vi "Load.vi"(8 "error in (no error)":errorcluster, 9 "Automatic?":bool, 10 "configuration file path":path, 11 "SettingsFile in":refnum<class "SettingsFile.lvclass">) -> (0 "error out":errorcluster, 3 "SettingsFile out":refnum<class "SettingsFile.lvclass">)   [LabVIEW 2018, in "SettingsFile.lvclass"]
uses:
  SettingsFile.lvclass
  SettingsFile.lvclass/SettingsFile.ctl
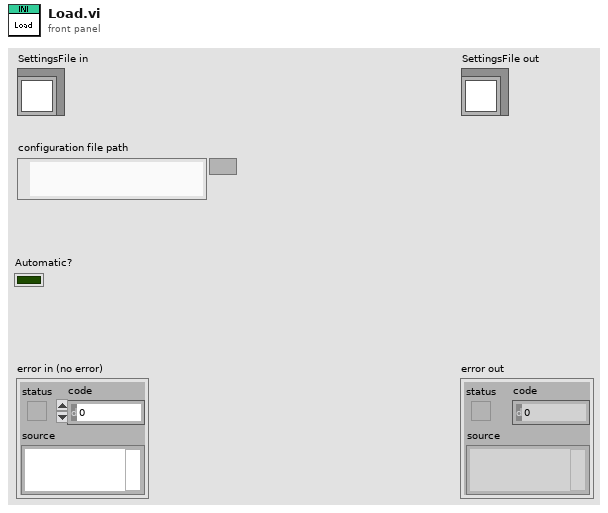
[diagram p1: front panel]
types:
  T1 = typedef "Graph_references.ctl" = cluster{"upper":T2, "lower":T2, "Freq graph":refnum<vi>, "Adaptive FF graph":refnum<vi>}
  T2 = typedef "graph_controls.ctl" = cluster{"Graph":refnum<vi>, "Time btn":refnum<vi>, "Amplitude btn":refnum<vi>, "Chart":refnum<vi>}
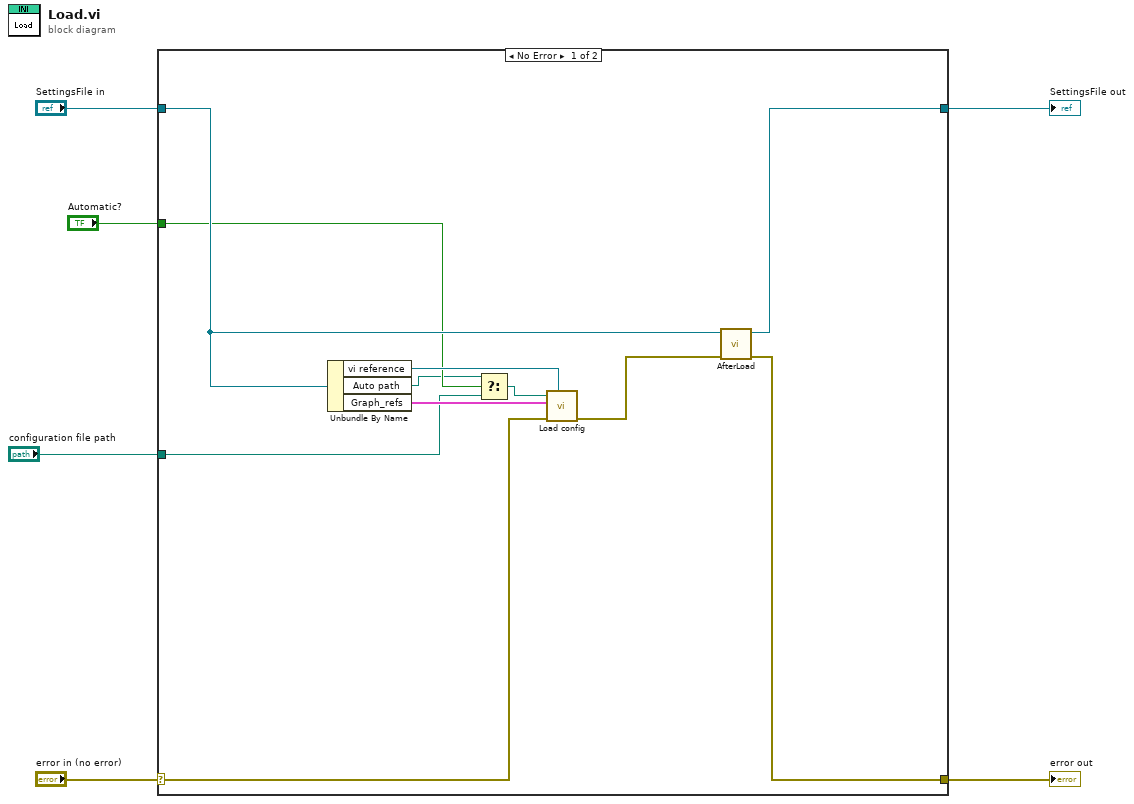
[diagram p0: block diagram]
diagram:
  n1 = case shown="No Error" "error in (no error)" {
    selector: "error in (no error)" -> [w15 w19]
    tunnel: [w11 w19] -> w5
    tunnel: [w12 w18] -> w3
    tunnel: "SettingsFile in" -> [w14 w18]
    tunnel: "Automatic?" -> [w10 _]
    tunnel: "configuration file path" -> [w8 _]
    frame No Error {
      n2 = Unbundle By Name(w14) -> ("vi reference"=w16:refnum<vi>, "Auto path"=w9:path, "Graph_refs"=w17:T1)
      n3 = Select(t=w9, s=w10, f=w8) -> (s? t:f=w7:path)
      n4 = call "Load config.vi"("Main VI"=w16, "error in (no error)"=w15, "Graph_refs"=w17, "configuration file path"=w7) -> ("error out"=w13:errorcluster)  [unwired: 7 in]
      n5 = call-dynamic "AfterLoad.vi"("error in (no error)"=w13, "SettingsFile in"=w14) -> ("error out"=w11:errorcluster, "SettingsFile out"=w12:refnum<class "SettingsFile.lvclass">)  [unwired: 8 in]
    }
    frame Error {
    }
  }
  "error out" <- w5
  "SettingsFile out" <- w3
